vi "电源管理UI - V1.vi"() -> ()   [LabVIEW 2016, in "PLC.lvlib"]
uses:
  PLC.lvlib
  <vilib>/Utility/miscctls.llb/LVPointTypeDef.ctl
panel:
  in  "多参数电源":bool
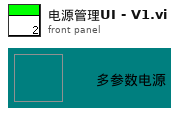
[diagram p1: front panel]
types:
  T1 = typedef "LVPointTypeDef.ctl" = cluster{"Horizontal":i16, "Vertical":i16}
  T2 = cluster{"命令":string, "DATA":cluster{"starting address":u16, "holding register value":u16}}
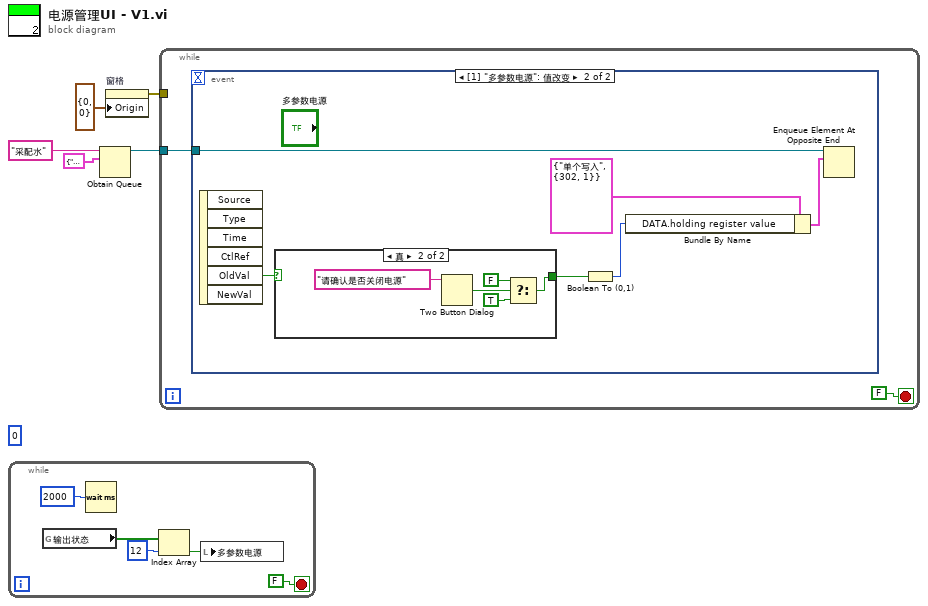
[diagram p0: block diagram]
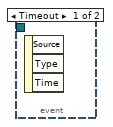
[diagram p2: hidden frame]
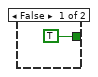
[diagram p3: hidden frame]
diagram:
  (unwired) u32 0 ("等待时间（毫秒）")
  n1 = while {
    stop <- FALSE stop-if-true
    n2 = global read "采配水全局变量.vi" "输出状态"() -> (w8:bool[])
    n3 = Wait (ms)(milliseconds to wait=u32 2000 ("等待时间（毫秒）")) -> ()  [unwired: 1 out]
    n4 = Index Array(array=w8, index=12 ("索引")) -> (element=w6:bool)
    n5 = local write "多参数电源"(w6) -> ()
  }
  n6 = Obtain Queue(name (unnamed)="采配水" ("名称（未命名）"), element data type=cluster{"命令":string, "数据":variant} {"命令"="", "数据"=variant}) -> (queue out=w1:refnum<queue>)  [unwired: 3 in, 2 out]
  n7 = property on="窗格" class="Pane"("Origin"=T1 {"Horizontal"=0, "Vertical"=0} ("原点")) -> (error out=w2:errorcluster)  [unwired: 2 in, 1 out]
  n8 = while {
    tunnel: w1 -> [w11]
    tunnel: w2 -> [_]
    stop <- FALSE stop-if-true
    n9 = event shown="[1] \"多参数电源\": 值改变" {
      selector: _ -> [_ _]
      dyn-events: _ -> [_ _]
      timeout: _ -> [_ _]
      tunnel: w11 -> [_ w16]
      event Timeout {
        n10 = event-data() -> ()  [unwired: 1 in, 3 out]
      }
      event "多参数电源": Value Change {
        n11 = event-data() -> ("OldVal"=w18:bool)  [unwired: 1 in, 5 out]
        n12 = case shown="真" w18 {
          tunnel: [TRUE ("T button?") w20] -> w17
          frame False {
          }
          frame True {
            n13 = Two Button Dialog(message="请确认是否关闭电源" ("消息")) -> (T button?=w23:bool)  [unwired: 2 in]
            n14 = Select(t=FALSE, s=w23, f=TRUE ("T button?")) -> (s? t:f=w20:bool)
          }
        }
        n15 = Boolean To (0,1)(Boolean=w17) -> (0, 1=w14:i16)
        n16 = Bundle By Name(cluster=T2 {"命令"="单个写入", "DATA"={"starting address"=302, "holding register value"=1}} ("元素"), "DATA.holding register value"=w14) -> (w13:T2)
        n17 = Enqueue Element At Opposite End(queue=w16, element=w13) -> ()  [unwired: 2 in, 3 out]
      }
    }
  }
